vi "Post-Build Action.vi"(5 "Files Generated by Build":path[](array[path]), 6 "Top Level/Always Included VIs":path[](array[path]), 7 "Destination Path":path, 8 "error in (no error)":errorcluster, 9 "Target Name":string, 10 "Build Specification Name":string, 11 "Project Path":path) -> (0 "error out":errorcluster)   [LabVIEW 2016, in "Script.lvlib"]
uses:
  Script.lvlib
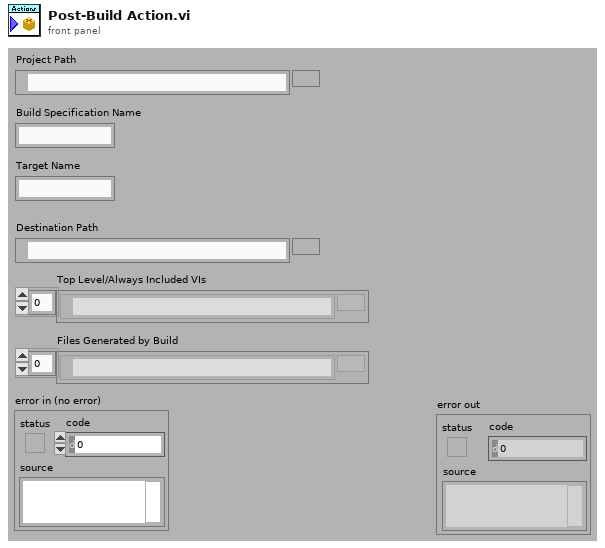
[diagram p1: front panel]
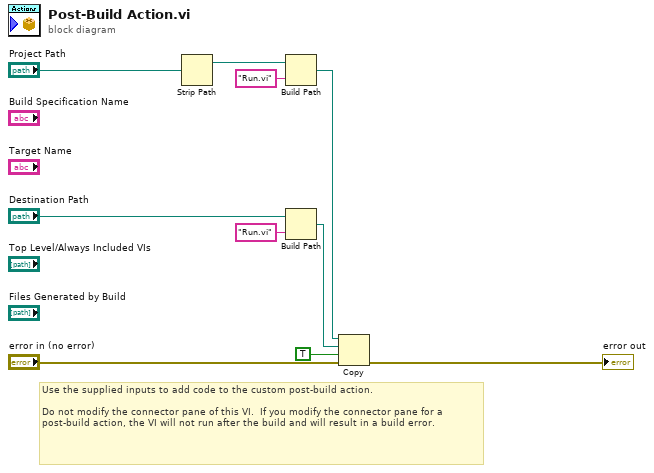
[diagram p0: block diagram]
diagram:
  # "Use the supplied inputs to add code to the custom post-build action.\n\nDo not modify the connector pane of this VI.  If you modify the connector pane for a post-build action, the VI will not run after the build and will result in a build error."
  n1 = Strip Path(path="Project Path") -> (stripped path=w9:path)  [unwired: 1 out]
  n2 = Build Path(base path=w9, name or relative path="Run.vi") -> (appended path=w3:path)
  n3 = Build Path(base path="Destination Path", name or relative path="Run.vi") -> (appended path=w2:path)
  n4 = Copy(8:"error in (no error)", 9:TRUE ("overwrite (F)"), 10:w2, 11:w3) -> (0:→"error out":errorcluster)  [unwired: 1 in, 2 out]
